vi "filter_images_by_phi.vi"(8 "Error In":errorcluster, 10 "Phi":dbl, 11 "Image Names":string[](array[string])) -> (0 "Error Out":errorcluster, 3 "Filtered Image Names":string[](array[string]))   [LabVIEW 2019]
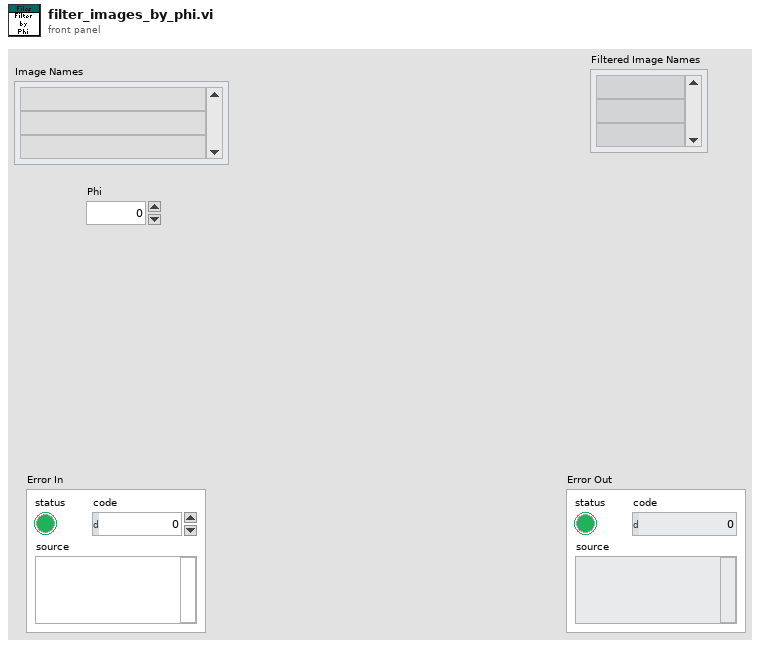
[diagram p1: front panel]
types:
  T1 = typedef "image_property_cluster_typedef.ctl" = cluster{"Stage Angle":dbl, "Sample Angle":dbl, "Polarizer 1 Angle":dbl, "Polarizer 2 Angle":dbl, "Sample Name":string}
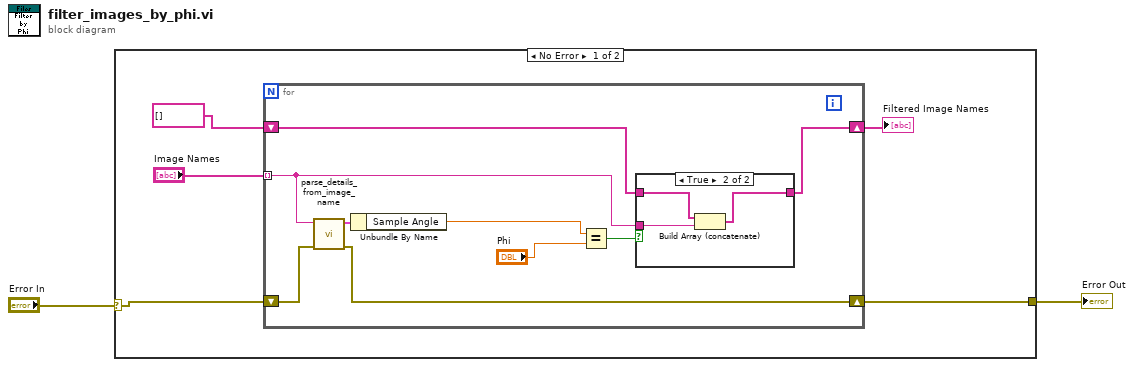
[diagram p0: block diagram]
diagram:
  n1 = case shown="No Error" "Error In" {
    selector: "Error In" -> [w6 w21]
    tunnel: [w5 w21] -> w1
    frame No Error {
      n2 = for {
        tunnel: "Image Names" -> [w11] mode=indexing
        shift-right: [w8] -> w5
        shift-left: w6 -> [w14]
        shift-right: [w10] -> w3
        shift-left: string[] [] -> [w12]
        n3 = call "parse_details_from_image_name.vi"("Error In"=w14, "Image Name"=w11) -> ("Error Out"=w8:errorcluster, "Image Properties"=w16:T1)  [unwired: 8 in]
        n4 = Unbundle By Name(w16) -> ("Sample Angle"=w15:dbl)
        n5 = Equal?(x=w15, y="Phi") -> (x = y?=w13:bool)
        n6 = case shown="True" w13 {
          tunnel: w12 -> [w17 w20]
          tunnel: w11 -> [_ w19]
          tunnel: [w17 w18] -> w10
          frame False {
          }
          frame True {
            n7 = Build Array (concatenate)(w20, w19) -> (w18:string[])
          }
        }
      }
      "Filtered Image Names" <- w3
    }
    frame Error {
    }
  }
  "Error Out" <- w1
